vi "Connect.vi"(8 "error in (no error)":errorcluster, 10 "Timeout":i32=10000, 11 "Sift Client in":refnum<class "Sift Client.lvclass">) -> (0 "error out":errorcluster, 2 "Success":bool, 3 "Sift Client out":refnum<class "Sift Client.lvclass">)   [LabVIEW 2024, in "Sift Client.lvlib" / "Sift Client.lvclass"]
doc: "Connect to Sift Proxy."
uses:
  Sift Client.lvclass
  Sift Client.lvclass/Sift Client.ctl
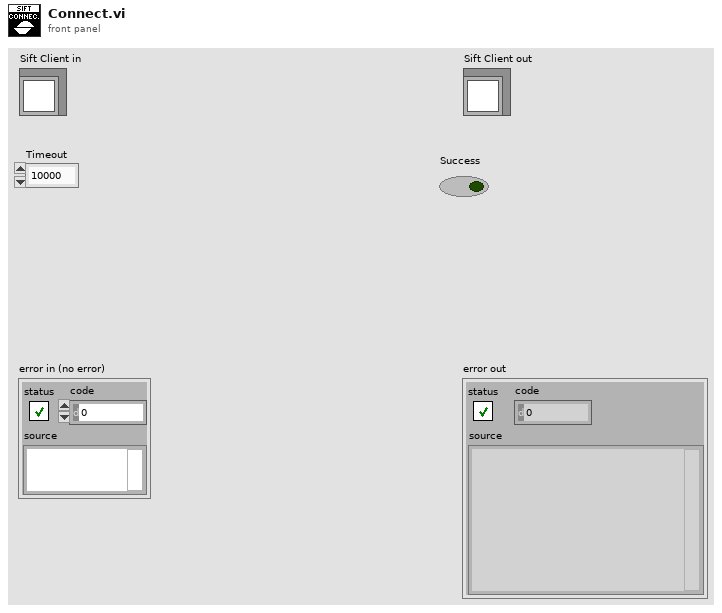
[diagram p1: front panel]
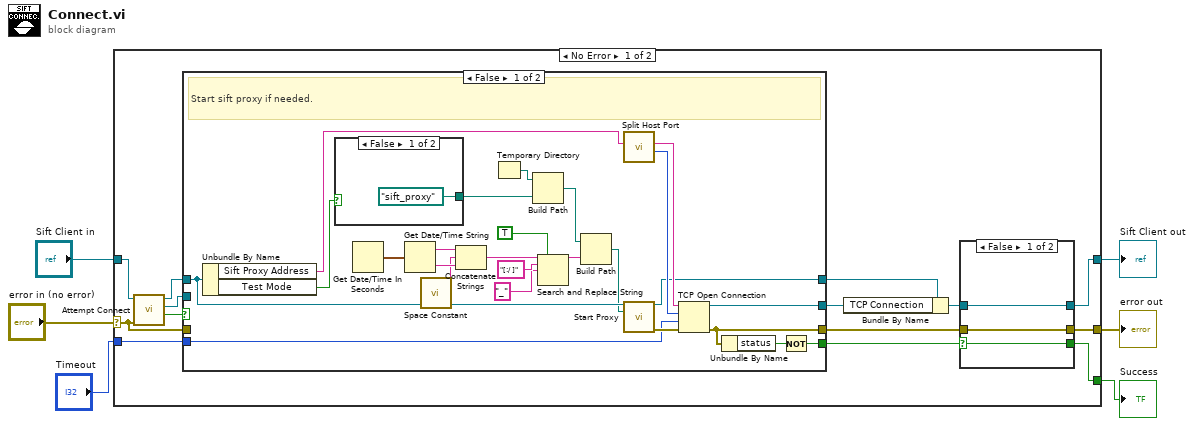
[diagram p0: block diagram]
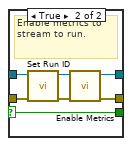
[diagram p2: hidden frame]
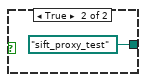
[diagram p3: hidden frame]
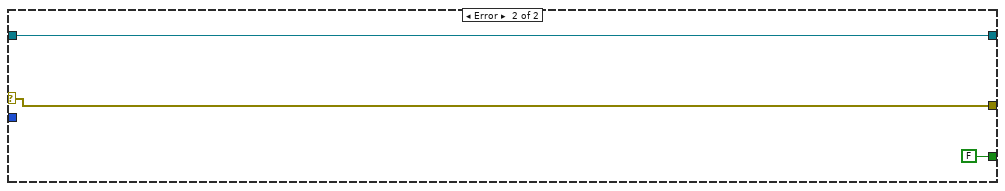
[diagram p5: hidden frame]
diagram:
  n1 = case shown="No Error" "error in (no error)" {
    selector: "error in (no error)" -> [w7 w64]
    tunnel: [w17 w64] -> w5
    tunnel: [w18 w63] -> w3
    tunnel: "Sift Client in" -> [w20 w63]
    tunnel: "Timeout" -> [w16 _]
    tunnel: [w8 FALSE] -> w1
    frame No Error {
      n2 = call-dynamic "Attempt Connect.vi"("error in (no error)"=w7, "Sift Client in"=w20) -> ("Success"=w9:bool, "Connection ID"=w10:refnum<k5>, "Sift Client out"=w19:refnum<class "Sift Client.lvclass">)  [unwired: 6 in, 1 out]
      n3 = case shown="False" w9 {
        selector: w9 -> [_ w59]
        tunnel: w19 -> [w42 w60]
        tunnel: w16 -> [w50 _]
        tunnel: [w49 w58] -> w15
        tunnel: [w48 w59] -> w14
        tunnel: [w41 w60] -> w13
        tunnel: [w47 w61] -> w12
        tunnel: w10 -> [_ w61]
        tunnel: w7 -> [_ w58]
        frame False {
          # "Start sift proxy if needed."
          n4 = Unbundle By Name(w42) -> ("Sift Proxy Address"=w53:string, "Test Mode"=w43:bool)
          n5 = case shown="False" w43 {
            tunnel: [path "sift_proxy" path "sift_proxy_test"] -> w45
            frame False {
            }
            frame True {
            }
          }
          n6 = Get Date/Time In Seconds() -> (seconds since 1Jan1904=w38:timestamp)
          n7 = Get Date/Time String(seconds (now)=w38) -> (date string=w39:string, time string=w33:string)  [unwired: 2 in]
          n8 = call <vilib>:"Space Constant.vi"() -> ("String"=w32:string)
          n9 = Concatenate Strings(w39, w32, w33) -> (w35:string)
          n10 = Temporary Directory() -> (w44:path)
          n11 = Build Path(base path=w44, name or relative path=w45) -> (appended path=w46:path)
          n12 = Search and Replace String(replace all?=TRUE, input string=w35, search string="[:/ ]", replace string="_" ("replace string (\"\")")) -> (result string=w31:string)  [unwired: 4 in, 3 out]
          n13 = Build Path(base path=w46, name or relative path=w31) -> (appended path=w40:path)
          n14 = call "Split Host Port.vi"("Address"=w53) -> ("Port"=w54:i32, "Hostname"=w55:string)  [unwired: 9 in]
          n15 = call-dynamic "Start Proxy.vi"("Sift Client in"=w42, "Storage Path"=w40) -> ("Sift Client out"=w41:refnum<class "Sift Client.lvclass">, "error out"=w51:errorcluster)  [unwired: 12 in]
          n16 = TCP Open Connection(address=w55, remote port or service name=w54, timeout ms (60000)=w50, error in (no error)=w51) -> (connection ID=w47:refnum<k5>, error out=w49:errorcluster)  [unwired: 1 in]
          n17 = Unbundle By Name(w49) -> ("status"=w52:bool)
          n18 = Not(x=w52) -> (.not. x?=w48:bool)
        }
        frame True {
          # "Connected successfully."
        }
      }
      n19 = Bundle By Name(cluster=w13, "TCP Connection"=w12) -> (w11:refnum<class "Sift Client.lvclass">)
      n20 = case shown="False" w14 {
        selector: w14 -> [w21 w24]
        tunnel: w11 -> [w23 w30]
        tunnel: w15 -> [w22 w28]
        tunnel: [w23 w26] -> w18
        tunnel: [w22 w25] -> w17
        tunnel: [w21 w24] -> w8
        frame False {
        }
        frame True {
          # "Enable metrics to stream to run."
          n21 = call-dynamic "Set Run ID.vi"("error in (no error)"=w28, "Sift Client in"=w30) -> ("error out"=w27:errorcluster, "Sift Client out"=w29:refnum<class "Sift Client.lvclass">)  [unwired: 8 in]
          n22 = call-dynamic "Enable Metrics.vi"("error in (no error)"=w27, "Sift Client in"=w29) -> ("error out"=w25:errorcluster, "Sift Client out"=w26:refnum<class "Sift Client.lvclass">)  [unwired: 8 in]
        }
      }
    }
    frame Error {
    }
  }
  "error out" <- w5
  "Sift Client out" <- w3
  "Success" <- w1
